vi "Error_Function.vi"(3 "output control":T1, 4 "data":variant, 5 "X":dbl[](array[numeric]), 6 "a":dbl[](array[numeric])) -> (0 "error out":errorcluster, 1 "f'(X,a)":dbl[][](array[numeric]), 2 "f(X,a)":dbl[](array[numeric]))   [LabVIEW 2012, in "DAQOrcaFlash.lvclass"]
doc: "This template is the starting point for creating a model function to be passed to the Nonlinear Curve Fit.vi."
uses:
  DAQOrcaFlash.lvclass
  <vilib>/gmath/NumericalOptimization/LM_output select.ctl
  <vilib>/gmath/NI_Gmath.lvlib
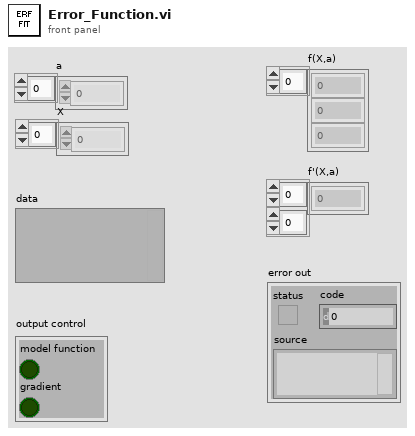
[diagram p1: front panel]
types:
  T1 = typedef "NI_Gmath.lvlib/LM_output select.ctl" = cluster{"model function":bool, "gradient":bool}
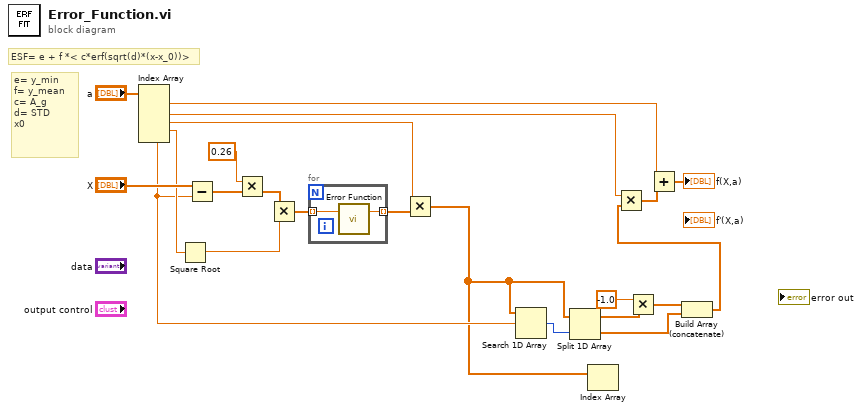
[diagram p0: block diagram]
diagram:
  # "e= y_min\nf= y_mean\nc= A_g\nd= STD\nx0"
  # "ESF= e + f *< c*erf(sqrt(d)*(x-x_0))>"
  n1 = Index Array(array="a") -> (element #1=w16:dbl, element #2=w15:dbl, element #3=w14:dbl, element #4=w13:dbl, element #5=w10:dbl)  [unwired: 5 in]
  n2 = Square Root(x=w13) -> (sqrt(x)=w19:dbl)
  n3 = Subtract(x="X", y=w10) -> (x-y=w7:dbl[])
  n4 = Multiply(x=0.26, y=w7) -> (x*y=w2:dbl[])
  n5 = Multiply(x=w2, y=w19) -> (x*y=w18:dbl[])
  n6 = for {
    tunnel: [w24] -> w20 mode=indexing
    tunnel: w18 -> [w23] mode=indexing
    n7 = call <vilib>:"Error Function.vi"("x"=w23) -> ("erf(x)"=w24:dbl)  [unwired: 2 in]
  }
  n8 = Multiply(x=w14, y=w20) -> (x*y=w4:dbl[])
  n9 = Search 1D Array(1D array=w4, element=w10) -> (index of element=w11:i32)  [unwired: 1 in]
  n10 = Split 1D Array(array=w4, index=w11) -> (first subarray=w9:dbl[], second subarray=w5:dbl[])
  n11 = Index Array(array=w4) -> ()  [unwired: 1 in, 1 out]
  n12 = Multiply(x=-1.0, y=w9) -> (x*y=w6:dbl[])
  n13 = Build Array (concatenate)(w6, w5) -> (w3:dbl[])
  n14 = Multiply(x=w15, y=w3) -> (x*y=w17:dbl[])
  n15 = Add(x=w16, y=w17) -> (x+y=→"f(X,a)":dbl[])
